vi "Master_ValueBuffer.vi"(10 "n":i32, 11 "new value":dbl) -> (3 "Last n values":dbl[](array[numeric]))   [LabVIEW 2017]
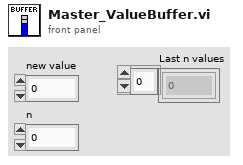
[diagram p1: front panel]
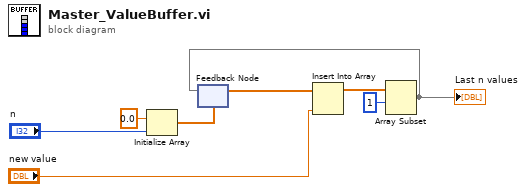
[diagram p0: block diagram]
diagram:
  n1 = Initialize Array(0.0 ("element"), "n") -> (w1:dbl[])
  n2 = feedback #1(w1) -> (w4:dbl[])
  n3 = Insert Into Array(array=w4, new element="new value") -> (w5:dbl[])  [unwired: 1 in]
  n4 = Array Subset(array=w5, index=1) -> (w7:dbl[])  [unwired: 1 in]
  "Last n values" <- w7
  n5 = feedback-in #1(w7) -> ()
